vi "part5.vi"() -> ()   [LabVIEW 2009]
panel:
  in  "stop":bool
  out "Array":bool[](array[boolean])
  # "Inputting from a 12 VDC source using an input module"
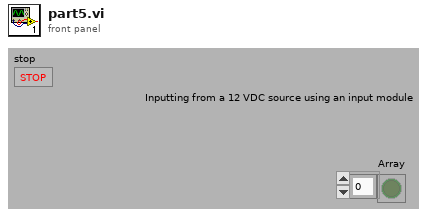
[diagram p1: front panel]
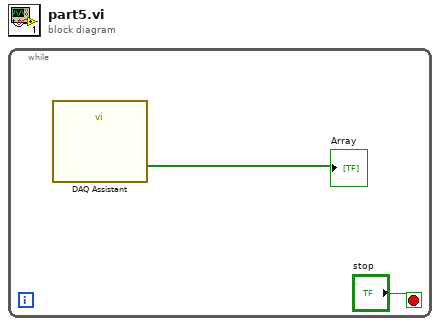
[diagram p0: block diagram]
diagram:
  n1 = while {
    stop <- "stop" stop-if-true
    n2 = call "DAQ Assistant"() -> ("data"=→"Array":bool[])  [unwired: 17 in, 2 out]
  }
